vi "Read Configuration.vi"(7 "Name":string, 8 "error in (no error)":errorcluster, 11 "Attribute.Config in":refnum<class "Attribute.Config.lvclass">) -> (0 "error out":errorcluster, 2 "Configuration":variant, 3 "Attribute.Config out":refnum<class "Attribute.Config.lvclass">)   [LabVIEW 2019, in "Attribute.Config.lvclass"]
doc: "JKI State Machine Objects (SMO) 1.3.0.56\nJKI - JKI\nCopyright (c) 2017, JKI"
uses:
  Attribute.Config.lvclass
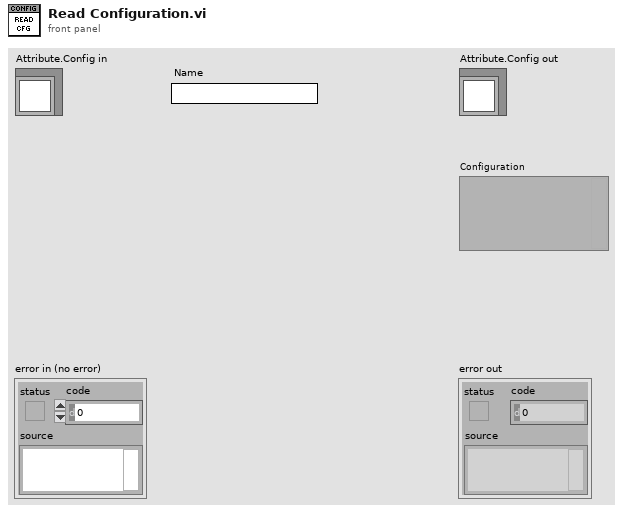
[diagram p1: front panel]
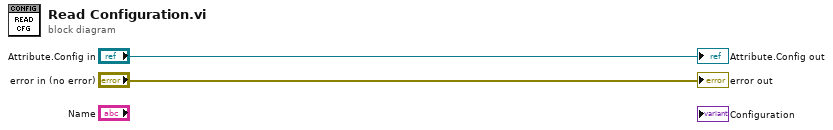
[diagram p0: block diagram]
diagram:
  "error out" <- "error in (no error)"
  "Attribute.Config out" <- "Attribute.Config in"
